vi "get_cube.vi"(11 "Path_image":path=path "C:/Users/swift/Desktop/Python/imec/Data/SKFX.300x300.Binning.2.frame.1.Gain.1.time.5.HDR-V6_corrected.hdr") -> (1 "IMAGE U8":u8[][][](array[numeric]), 3 "CUBE":sgl[][][](array[numeric]))   [LabVIEW 2018]
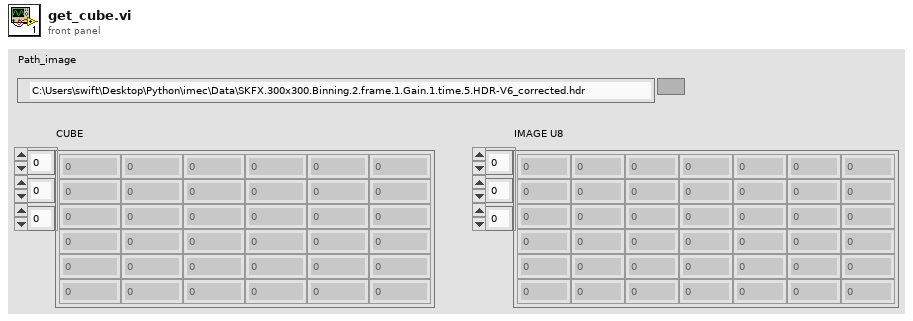
[diagram p1: front panel]
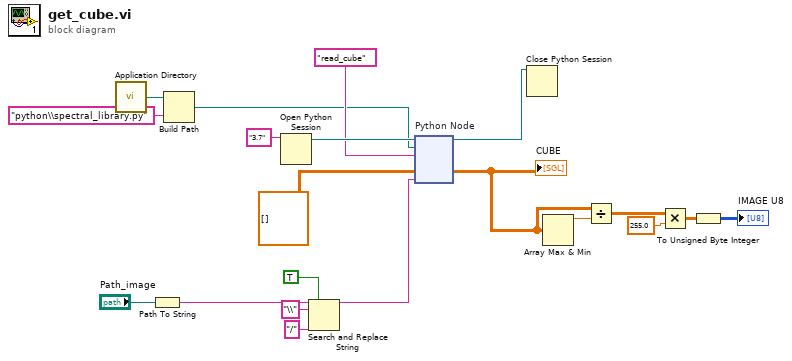
[diagram p0: block diagram]
diagram:
  n1 = call <vilib>:"Application Directory.vi"() -> ("Application Directory"=w10:path)
  n2 = Path To String(path="Path_image") -> (string=w19:string)
  n3 = Build Path(base path=w10, name or relative path="python\\spectral_library.py" ("nom ou chemin relatif")) -> (appended path=w8:path)
  n4 = Open Python Session(python version="3.7" ("Python version")) -> (session out=w14:refnum<k35>)  [unwired: 2 in, 1 out]
  n5 = Search and Replace String(replace all?=TRUE ("replace all? (F)"), input string=w19, search string="\\", replace string="/" ("replace string (\"\")")) -> (result string=w11:string)  [unwired: 4 in, 3 out]
  n6 = node "Python Node"(w14, w8, "read_cube" ("function name"), sgl[][][] [], w11) -> (w1:refnum<k35>, w3:sgl[][][])  [unwired: 2 in, 3 out]
  "CUBE" <- w3
  n7 = Close Python Session(session in=w1) -> ()  [unwired: 1 in, 1 out]
  n8 = Array Max & Min(array=w3) -> (max value=w7:sgl)  [unwired: 3 out]
  n9 = Divide(x=w3, y=w7) -> (x/y=w5:sgl[][][])
  n10 = Multiply(x=w5, y=sgl 255.0) -> (x*y=w4:sgl[][][])
  n11 = To Unsigned Byte Integer(number=w4) -> (unsigned 8bit integer=→"IMAGE U8":u8[][][])
